vi "Read Measurement 2 Channels.vi"(5 "Channel 1 (1: Channel 1)":i32(ring)=1 items=["Channel 1"=1, "Channel 2"=2, "Channel 3"=3, "Channel 4"=4], 7 "Channel 2 (2: Channel 2)":i32(ring)=2 items=["Channel 1"=1, "Channel 2"=2, "Channel 3"=3, "Channel 4"=4], 8 "error in (no error)":errorcluster, 10 "VISA resource name":refnum<visa-resource-name>, 11 "Osciloscope in":refnum<class "Osciloscope.lvclass">) -> (0 "error out":errorcluster, 2 "VISA resource name out":refnum<visa-resource-name>, 3 "Osciloscope out":refnum<class "Osciloscope.lvclass">, 4 "Measurement":dbl, 6 "Units":string)   [LabVIEW 2020, in "Controlador.lvlib" / "Osciloscope.lvclass"]
uses:
  Osciloscope.lvclass
  <instrlib>/Tektronix TDS 200 1000 2000 Series/Tektronix TDS 200 1000 2000 Series.lvlib
panel:
  in  "Measurement Type (0: Phase)":i32(ring) items=["Phase", "Delay", "DelayRR", "DelayRF", "DelayFR", "DelayFF"]
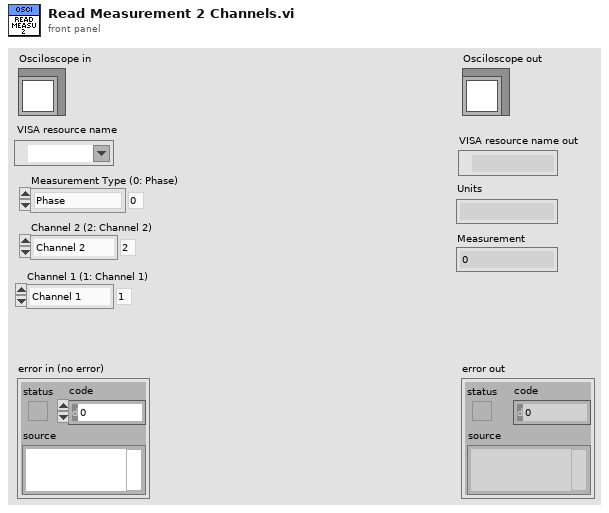
[diagram p1: front panel]
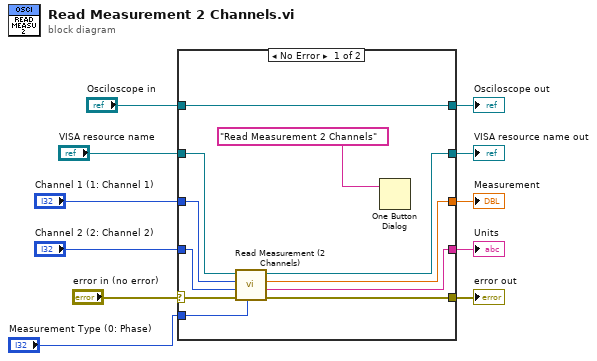
[diagram p0: block diagram]
diagram:
  n1 = case shown="No Error" "error in (no error)" {
    selector: "error in (no error)" -> [w21 w24]
    tunnel: [w20 w24] -> w10
    tunnel: [w22 w23] -> w8
    tunnel: "Osciloscope in" -> [w22 w23]
    tunnel: "VISA resource name" -> [w19 _]
    tunnel: "Channel 1 (1: Channel 1)" -> [w18 _]
    tunnel: "Channel 2 (2: Channel 2)" -> [w17 _]
    tunnel: "Measurement Type (0: Phase)" -> [w16 _]
    tunnel: [w15 _] -> w3
    tunnel: [w14 _] -> w2
    tunnel: [w13 _] -> w1
    frame No Error {
      n2 = call <instrlib>:"Read Measurement (2 Channels).vi"("Measurement Type (0: Phase)"=w16, "error in (no error)"=w21, "Channel 2 (2: Channel 2)"=w17, "Channel 1 (1: Channel 1)"=w18, "VISA resource name"=w19) -> ("error out"=w20:errorcluster, "Units"=w13:string, "Measurement"=w14:dbl, "VISA resource name out"=w15:refnum<visa-resource-name>)  [unwired: 3 in]
      n3 = One Button Dialog(message="Read Measurement 2 Channels") -> ()  [unwired: 1 in, 1 out]
    }
    frame Error {
    }
  }
  "error out" <- w10
  "Osciloscope out" <- w8
  "Units" <- w1
  "Measurement" <- w2
  "VISA resource name out" <- w3
